vi "CANOpen_Load 9881 Bitfile.vi"(8 "error in (no error)":errorcluster, 11 "Item Ref in":T1 format="%.0x") -> (0 "error out":errorcluster, 2 "FPGA Session":u32, 3 "Item Ref out":T1=18446744073709551615 format="%.0x")   [LabVIEW 2021, in "CANOpen Addon Engine.lvlib"]
uses:
  CANOpen Addon Engine.lvlib
  <vilib>/NI VeriStand/Custom Device API/Custom Device Item Ref.ctl
  Shared/CANOpen Addon GUID Lookup Global.vi
  <vilib>/NI VeriStand/Custom Device API/Get Item Property (Variant).vi
  <vilib>/NI VeriStand/Custom Device API/Get Item Property (Path).vi
  Shared/CANOpen Addon Shared.lvlib
  <vilib>/NI VeriStand/Custom Device API/Custom Device API.lvlib
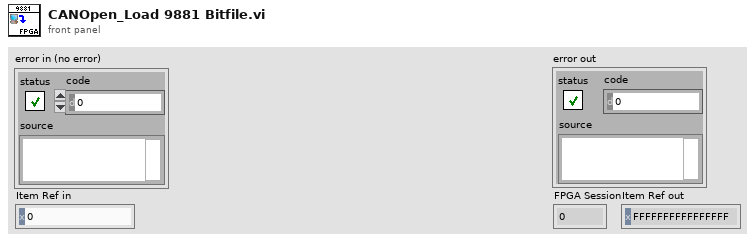
[diagram p1: front panel]
types:
  T1 = typedef "Custom Device API.lvlib/Custom Device Item Ref.ctl" = u64
  T2 = typedef "CANOpen Addon Shared.lvlib/CANOpen_Bus Settings.ctl" = cluster{"CANOpen Interface Name":T3, "Baud Rate":T4, "Termination":bool, "Sync Period (ms)":i64, "Enable 9881":bool, "RIO Device":u16, "Enable SYNC":bool, "Scan & Print":bool}
  T3 = typedef "CANOpen Addon Shared.lvlib/CANOpen Interface Name.ctl" = u32
  T4 = typedef "CANopen BaudRate.ctl" = u32
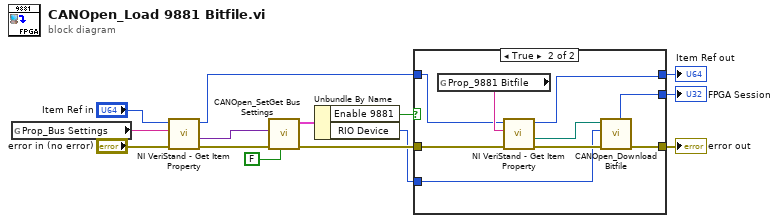
[diagram p0: block diagram]
diagram:
  n1 = global read "CANOpen Addon GUID Lookup Global.vi" "Prop_Bus Settings"() -> (w14:string)
  n2 = call-poly <vilib>:"NI VeriStand - Get Item Property.vi"("error in (no error)"="error in (no error)", "Property Name"=w14, "Item Ref in"="Item Ref in") -> ("error out"=w13:errorcluster, "Value"=w12:variant, "Item Ref out"=w11:T1)  [unwired: 5 in, 1 out]
  n3 = call "CANOpen_SetGet Bus Settings.vi"("Set Parameters"=FALSE, "error in (no error)"=w13, "Parameters"=w12) -> ("error out"=w10:errorcluster, "CANOpen Bus Settings"=w9:T2)  [unwired: 6 in, 1 out]
  n4 = Unbundle By Name(w9) -> ("Enable 9881"=w8:bool, "RIO Device"=w3:u16)
  n5 = case shown="True" w8 {
    tunnel: w11 -> [w15 w22]
    tunnel: w10 -> [w16 w21]
    tunnel: [w16 w20] -> w7
    tunnel: [_ w19] -> w4
    tunnel: w3 -> [_ w18]
    tunnel: [w15 w17] -> w2
    frame False {
    }
    frame True {
      n6 = global read "CANOpen Addon GUID Lookup Global.vi" "Prop_9881 Bitfile"() -> (w25:string)
      n7 = call-poly <vilib>:"NI VeriStand - Get Item Property.vi"("error in (no error)"=w21, "Property Name"=w25, "Item Ref in"=w22) -> ("error out"=w24:errorcluster, "Value"=w23:path, "Item Ref out"=w17:T1)  [unwired: 5 in, 1 out]
      n8 = call "CANOpen_Download Bitfile.vi"("error in (no error)"=w24, "Port data.RIO device address"=w18, "path"=w23) -> ("error out"=w20:errorcluster, "FPGA Session"=w19:u32)  [unwired: 7 in]
    }
  }
  "error out" <- w7
  "FPGA Session" <- w4
  "Item Ref out" <- w2
